vi "resetSelection.vi"(8 "error in (no error)":errorcluster, 10 "Selection":i32=-1, 11 "AbstractMultiColumnListBoxAdapter in":refnum<class "AbstractMultiColumnListBoxAdapter.lvclass">) -> (0 "error out":errorcluster, 3 "AbstractMultiColumnListBoxAdapter out":refnum<class "AbstractMultiColumnListBoxAdapter.lvclass">)   [LabVIEW 2020, in "AbstractMultiColumnListBoxAdapter.lvclass"]
uses:
  AbstractMultiColumnListBoxAdapter.lvclass
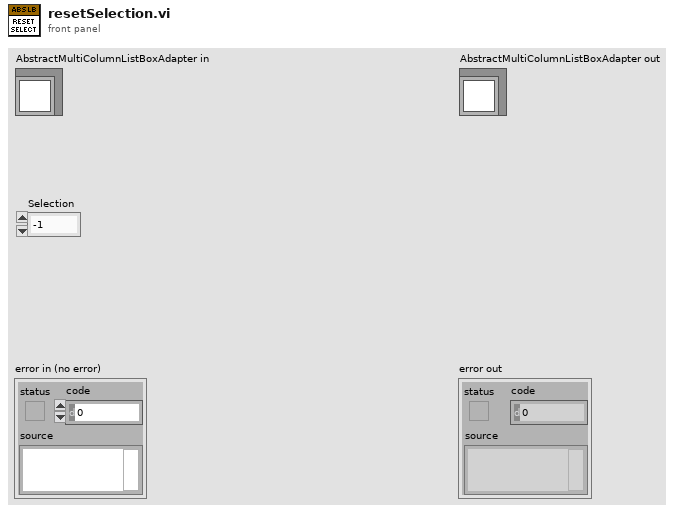
[diagram p1: front panel]
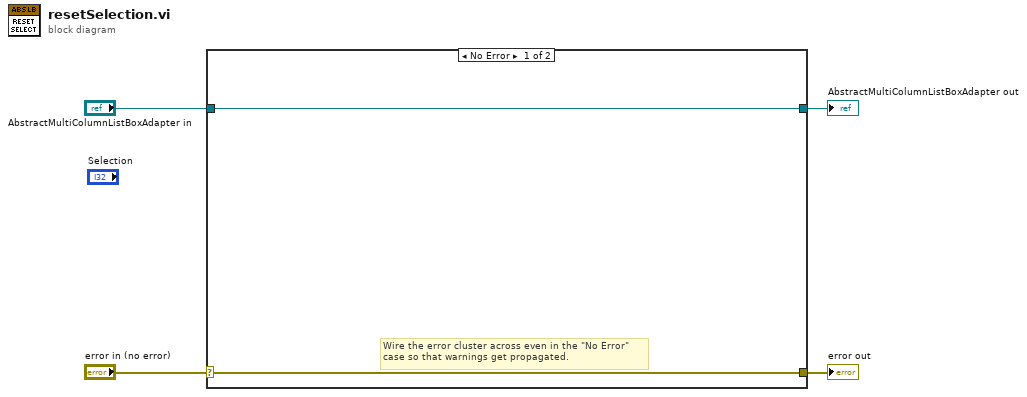
[diagram p0: block diagram]
diagram:
  n1 = case shown="No Error" "error in (no error)" {
    selector: "error in (no error)" -> [w5 w8]
    tunnel: [w5 w8] -> w3
    tunnel: [w6 w7] -> w1
    tunnel: "AbstractMultiColumnListBoxAdapter in" -> [w6 w7]
    frame No Error {
      # "Wire the error cluster across even in the \"No Error\"\ncase so that warnings get propagated."
    }
    frame Error {
    }
  }
  "error out" <- w3
  "AbstractMultiColumnListBoxAdapter out" <- w1
